vi "FaceTrackingLbvnew.vi"() -> ()   [LabVIEW 2012]
uses:
  <userlib>/ImageProcessing/InitCamera_NTSC.vi
  <userlib>/ImageProcessing/LV86_Morph_Erosion.vi
  <userlib>/ImageProcessing/LV86_Morph_Dilation.vi
  <userlib>/ImageProcessing/LV86_Morph_Close.vi
panel:
  out "?":picture
  out "x/y":dbl
  out "Area2":dbl
  out "Hight":dbl
  out "Width":dbl
  out "Area":dbl
  out "0's coun t":dbl
  out "Dif":picture
  out "image":picture
  in  "Boolean":bool
  out "Before Morphology":picture
  out "After Morphology":picture
  in  "Cb":cluster{i32, i32}(slide)={0, 3} scale=0.0..255.0
  in  "Cr":cluster{i32, i32}(slide)={0, 3} scale=0.0..255.0
  out "Cr":dbl[](array[numeric])
  out "Cb":dbl[](array[numeric])
  out "Y":dbl[](array[numeric])
  out "Original":picture
  in  "Stop":bool
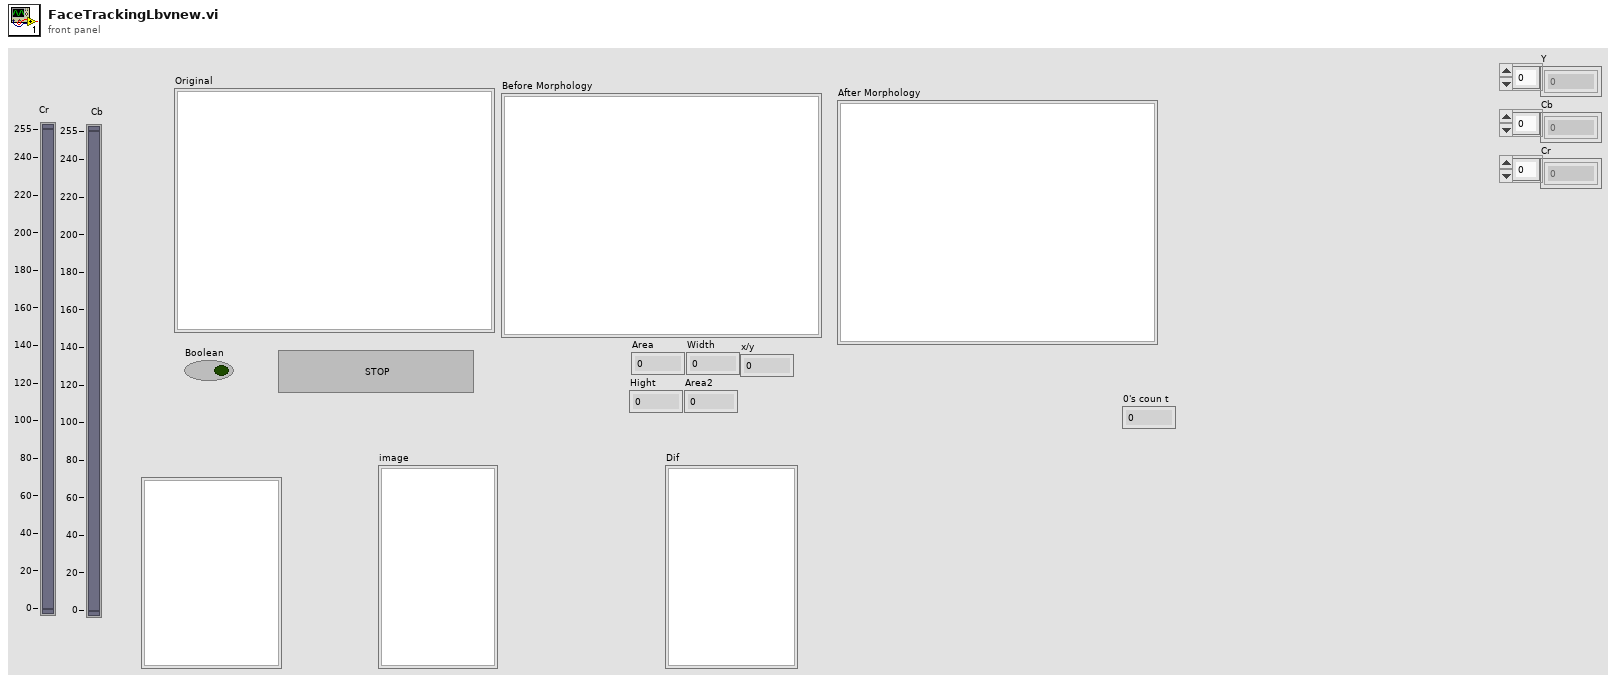
[diagram p1: front panel]
types:
  T1 = typedef "QT_Ref.ctl" = refnum<k1>
  T2 = cluster{"left":i16, "top":i16, "right":i16, "bottom":i16}
  T3 = typedef "QT_Image.ctl" = cluster{"Width":i32, "Height":i32, "Depth":i32, "data":u8[], "Compressed data":u8[], "Color table":u32[], "Duration":i32, "Options":i32, "Timestamp":i32, "ID":i32, "Reserved":i32, "Dialogs":u32}
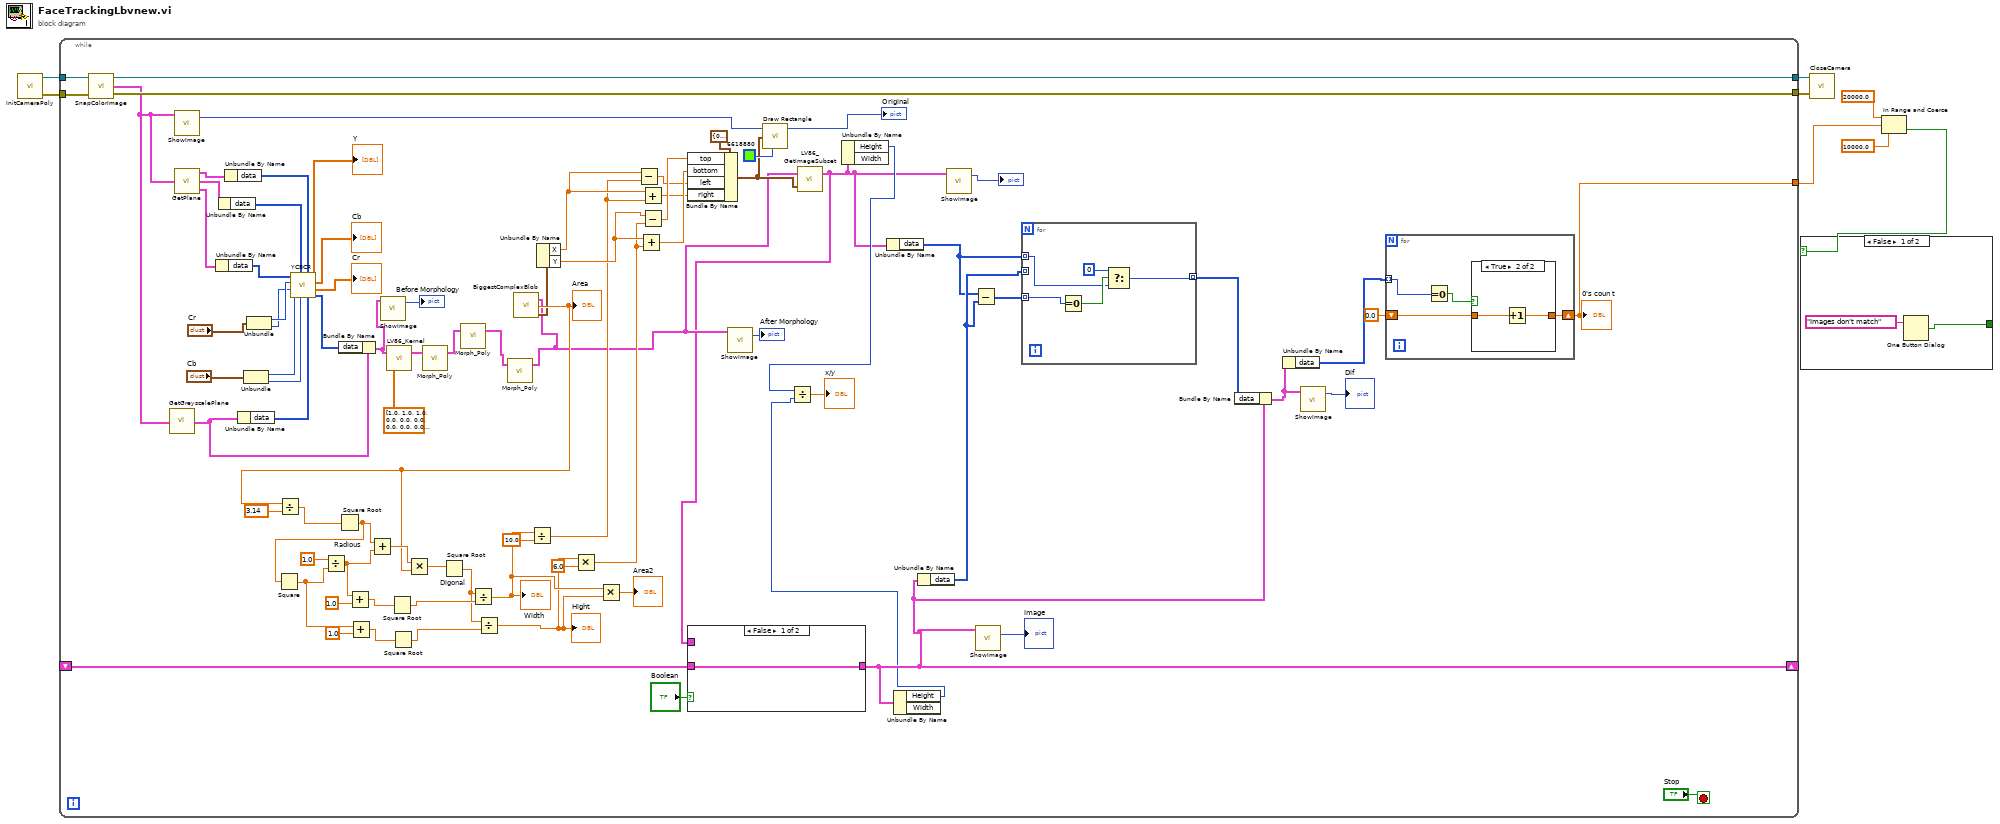
[diagram p0: block diagram]
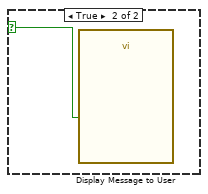
[diagram p2: hidden frame]
diagram:
  n1 = call-poly <userlib>:"InitCameraPoly.vi"() -> ("error out"=w5:errorcluster, "QT Ref Out"=w6:T1)  [unwired: 2 in]
  n2 = while {
    tunnel: w5 -> [w93]
    tunnel: w6 -> [w92]
    tunnel: [w91] -> w7
    tunnel: [w90] -> w8
    shift-right: [w14] -> _
    shift-left: _ -> [w48]
    tunnel: [w58] -> w4
    stop <- "Stop" stop-if-true
    n3 = call <userlib>:"SnapColorImage.vi"("error in (no error)"=w93, "QT Ref In"=w92) -> ("error out"=w91:errorcluster, "Image Out"=w66:T3, "QT Ref Out"=w90:T1)  [unwired: 1 in]
    n4 = call <userlib>:"GetGreyscalePlane.vi"("Image In"=w66) -> ("Greyscale  Out"=w69:T3)
    n5 = call <userlib>:"ShowImage.vi"("Image"=w66) -> ("image"=w36:picture)  [unwired: 2 in, 1 out]
    n6 = call <userlib>:"GetPlane.vi"("Image In"=w66) -> ("Blue Plane Out"=w86:T3, "Green Plane Out"=w87:T3, "Red Plane Out"=w88:T3)
    n7 = Unbundle By Name(w86) -> ("data"=w76:u8[])
    n8 = Unbundle By Name(w87) -> ("data"=w80:u8[])
    n9 = Unbundle By Name(w88) -> ("data"=w77:u8[])
    n10 = Unbundle By Name(w69) -> ("data"=w70:u8[])
    n11 = Unbundle("Cb") -> (w82:i32, w78:i32)
    n12 = Unbundle("Cr") -> (w85:i32, w84:i32)
    n13 = call "YCBCR.vi"("data 3"=w70, "data"=w77, "Numeric"=w78, "data 2"=w80, "Numeric 2"=w82, "Numeric 3"=w84, "Numeric 4"=w85, "data 4"=w76) -> ("Array"=w71:u8[], "Cr"=→"Cr":dbl[], "Cb"=→"Cb":dbl[], "Y"=→"Y":dbl[])
    n14 = Bundle By Name(cluster=w69, "data"=w71) -> (w28:T3)
    n15 = call <userlib>:"ShowImage.vi"("Image"=w28) -> ("image"=→"Before Morphology":picture)  [unwired: 2 in, 1 out]
    n16 = call <userlib>:"LV86_Kernel.vi"("Kernel"=sgl[][] [[1.0, 1.0, 1.0, 0.0, 0.0, 0.0, 0.0, 0.0, 0.0, 0.0], [1.0, 1.0, 1.0, 0.0, 0.0, 0.0, 0.0, 0.0, 0.0, 0.0], [1.0, 1.0, 1.0, 0.0, 0.0, 0.0, 0.0, 0.0, 0.0, 0.0], [0.0, 0.0, 0.0, 1.0, 0.0, 0.0, 0.0, 0.0, 0.0, 0.0], [0.0, 0.0, 0.0, 0.0, 0.0, 0.0, 0.0, 0.0, 0.0, 0.0], [0.0, 0.0, 0.0, 0.0, 0.0, 0.0, 0.0, 0.0, 0.0, 0.0], [0.0, 0.0, 0.0, 0.0, 0.0, 0.0, 0.0, 0.0, 0.0, 0.0], [0.0, 0.0, 0.0, 0.0, 0.0, 0.0, 0.0, 0.0, 0.0, 0.0], [0.0, 0.0, 0.0, 0.0, 0.0, 0.0, 0.0, 0.0, 0.0, 0.0], [0.0, 0.0, 0.0, 0.0, 0.0, 0.0, 0.0, 0.0, 0.0, 1.0]], "Image in"=w28) -> ("Image out"=w27:T3)  [unwired: 1 in]
    n17 = call-poly <userlib>:"Morph_Poly.vi"("Image in"=w27) -> ("Image out"=w26:T3)  [unwired: 2 in]
    n18 = call-poly <userlib>:"Morph_Poly.vi"("Image in"=w26) -> ("Image out"=w25:T3)  [unwired: 2 in]
    n19 = call-poly <userlib>:"Morph_Poly.vi"("Image in"=w25) -> ("Image out"=w15:T3)  [unwired: 2 in]
    n20 = call <userlib>:"BiggestComplexBlob.vi"("Image in"=w15) -> ("Centroid"=w35:cluster{"X":dbl, "Y":dbl}, "Area"=w50:dbl)  [unwired: 1 in, 1 out]
    "Area" <- w50
    n21 = Divide(x=w50, y=3.14) -> (x/y=w54:dbl)
    n22 = Square Root "Radious"(x=w54) -> (sqrt(x)=w52:dbl)
    n23 = Square(x=w52) -> (x^2=w42:dbl)
    n24 = Divide(x=1.0, y=w42) -> (x/y=w47:dbl)
    n25 = Add(x=w47, y=1.0) -> (x+y=w45:dbl)
    n26 = Add(x=w42, y=1.0) -> (x+y=w40:dbl)
    n27 = Add(x=w52, y=w47) -> (x+y=w51:dbl)
    n28 = Square Root(x=w45) -> (sqrt(x)=w44:dbl)
    n29 = Square Root(x=w40) -> (sqrt(x)=w39:dbl)
    n30 = Multiply(x=w51, y=w50) -> (x*y=w49:dbl)
    n31 = Square Root "Digonal"(x=w49) -> (sqrt(x)=w43:dbl)
    n32 = Divide(x=w43, y=w44) -> (x/y=w21:dbl)
    "Width" <- w21
    n33 = Divide(x=w43, y=w39) -> (x/y=w19:dbl)
    "Hight" <- w19
    n34 = Divide(x=w21, y=10.0) -> (x/y=w22:dbl)
    n35 = Unbundle By Name(w35) -> ("X"=w23:dbl, "Y"=w24:dbl)
    n36 = Multiply(x=w19, y=6.0) -> (x*y=w17:dbl)
    n37 = Multiply(x=w21, y=w19) -> (x*y=→"Area2":dbl)
    n38 = Subtract(x=w23, y=w22) -> (x-y=w31:dbl)
    n39 = Add(x=w24, y=w17) -> (x+y=w34:dbl)
    n40 = Add(x=w23, y=w22) -> (x+y=w32:dbl)
    n41 = Subtract(x=w24, y=w17) -> (x-y=w33:dbl)
    n42 = Bundle By Name(cluster=T2 {"left"=0, "top"=0, "right"=0, "bottom"=0} ("rect"), "top"=w33, "bottom"=w34, "left"=w31, "right"=w32) -> (w16:T2)
    n43 = call <userlib>:"ShowImage.vi"("Image"=w15) -> ("image"=→"After Morphology":picture)  [unwired: 2 in, 1 out]
    n44 = call <vilib>:"Draw Rectangle.vi"("picture"=w36, "rect"=w16, "color(black)"=u32 6618880) -> ("new picture"=→"Original":picture)  [unwired: 6 in]
    n45 = call <userlib>:"LV86_GetImageSubset.vi"("ROI"=w16, "Image In"=w15) -> ("Image out"=w9:T3)  [unwired: 1 in]
    n46 = case shown="False" "Boolean" {
      tunnel: w9 -> [_ w102]
      tunnel: [w101 w102] -> w14
      tunnel: w48 -> [w101 _]
      frame False {
      }
      frame True {
      }
    }
    n47 = Unbundle By Name(w9) -> ("Height"=w13:i32)  [unwired: 1 out]
    n48 = Unbundle By Name(w9) -> ("data"=w57:u8[])
    n49 = Unbundle By Name(w14) -> ("Height"=w12:i32)  [unwired: 1 out]
    n50 = Divide(x=w13, y=w12) -> (x/y=→"x/y":dbl)
    n51 = Unbundle By Name(w14) -> ("data"=w63:u8[])
    n52 = call <userlib>:"ShowImage.vi"("Image"=w9) -> ("image"=→"?":picture)  [unwired: 2 in, 1 out]
    n53 = Subtract(x=w57, y=w63) -> (x-y=w73:u8[])
    n54 = call <userlib>:"ShowImage.vi"("Image"=w14) -> ("image"=→"image":picture)  [unwired: 2 in, 1 out]
    n55 = for {
      tunnel: w73 -> [w107] mode=indexing
      tunnel: w63 -> [_] mode=indexing
      tunnel: w57 -> [w103] mode=indexing
      tunnel: [w105] -> w72 mode=indexing
      n56 = Equal To 0?(x=w107) -> (x = 0?=w106:bool)
      n57 = Select(t=u8 0, s=w106, f=w103) -> (s? t:f=w105:u8)
    }
    n58 = Bundle By Name(cluster=w14, "data"=w72) -> (w61:T3)
    n59 = Unbundle By Name(w61) -> ("data"=w60:u8[])
    n60 = call <userlib>:"ShowImage.vi"("Image"=w61) -> ("image"=→"Dif":picture)  [unwired: 2 in, 1 out]
    n61 = for {
      tunnel: w60 -> [w97] mode=indexing
      shift-right: [w95] -> w58
      shift-left: 0.0 -> [w94]
      n62 = Equal To 0?(x=w97) -> (x = 0?=w96:bool)
      n63 = case shown="True" w96 {
        tunnel: [w98 w100] -> w95
        tunnel: w94 -> [w98 w99]
        frame False {
        }
        frame True {
          n64 = Increment(x=w99) -> (x+1=w100:dbl)
        }
      }
    }
    "0's coun t" <- w58
  }
  n65 = call <userlib>:"CloseCamera.vi"("error in (no error)"=w7, "QT Ref In"=w8) -> ()  [unwired: 1 in, 1 out]
  n66 = In Range and Coerce(upper limit=20000.0, x=w4, lower limit=10000.0) -> (In Range?=w1:bool)  [unwired: 1 out]
  n67 = case shown="False" w1 {
    selector: w1 -> [_ w110]
    tunnel: [w109 _] -> _
    frame False {
      n68 = One Button Dialog(message="Images don't match") -> (true=w109:bool)  [unwired: 1 in]
    }
    frame True {
      n69 = call "Display Message to User"("Enable"=w110) -> ()  [unwired: 9 in, 2 out]
    }
  }
